vi "读取发送表.vi"() -> (2 "输入数组":string[][](array[string]))   [LabVIEW 2016]
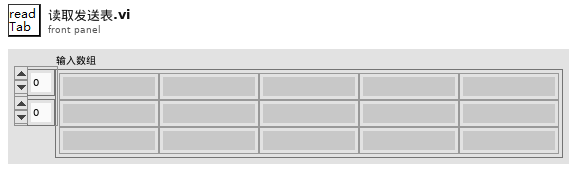
[diagram p1: front panel]
types:
  T1 = enum16{"open", "replace", "create", "open or create", "replace or create", "replace or create with confirmation"}
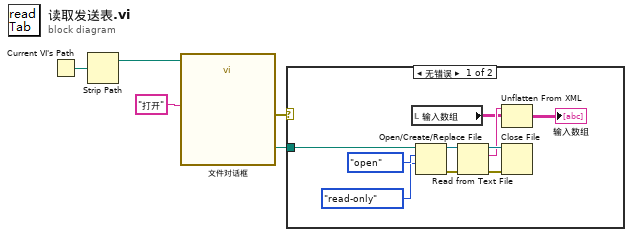
[diagram p0: block diagram]
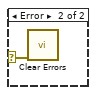
[diagram p2: hidden frame]
diagram:
  n1 = Current VI's Path() -> (path=w5:path)
  n2 = Strip Path(path=w5) -> (stripped path=w1:path)  [unwired: 1 out]
  n3 = call "文件对话框"("start path"=w1, "button label"="打开") -> ("selected path"=w3:path, "error out"=w2:errorcluster)  [unwired: 10 in, 2 out]
  n4 = case shown="无错误" w2 {
    selector: w2 -> [_ w16]
    tunnel: w3 -> [w15 _]
    frame No Error {
      n5 = local read "输入数组"() -> (w6:string[][])
      n6 = Open/Create/Replace File(file path (use dialog)=w15, operation (0:open)=T1."open" ("操作(0:open)"), access (0:read/write)=enum16{"read/write", "read-only", "write-only"}."read-only" ("权限(0:read/write)")) -> (refnum out=w12:refnum<file>, error out=w11:errorcluster)  [unwired: 3 in, 1 out]
      n7 = Read from Text File(file (use dialog)=w12, error in=w11) -> (refnum out=w10:refnum<file>, text=w8:string, error out=w9:errorcluster)  [unwired: 2 in, 1 out]
      n8 = Unflatten From XML(xml string=w8, type=w6) -> (value=→"输入数组":string[][])  [unwired: 1 in, 1 out]
      n9 = Close File(refnum=w10, error in=w9) -> ()  [unwired: 2 out]
    }
    frame Error {
      n10 = call <vilib>:"Clear Errors.vi"("error in (no error)"=w16) -> ()  [unwired: 5 in, 2 out]
    }
  }
